vi "PSTR-Save Data.vi"(0 "Data in":T12, 1 "PSTR Params":T4={"Stimulus"={"Ear"=enum."Right", "BW (oct)"=0.25, "Seed"=37, "Ramp (ms)"=5.0, "On time (ms)"=300.0, "Off time (ms)"=300.0, "Delay (ms)"=10000.0}, "FreqSeq"={"Min (kHz)"=4.0, "Max (kHz)"=64.0, "Step (oct)"=0.5}, "LevelSeq"={"Min (dB)"=0.0, "Max (dB)"=80.0, "Step (dB)"=20.0}, "Seq"={"Order"=enum."Sequential", "Averages"=20}, "Response"={"Grass gain"=10000.0, "Window (ms)"=0.0}, "Hidden"={"Sample rate (Hz)"=200000.0, "Nfft"=0, "save raw"=FALSE, "sep"=0.0, "Window"=enum."NONE"}, "RejThr"=0.0}, 2 "Expt State":T1, 5 "path":path, 7 "CFTS-PSTR":T3, 11 "error in":errorcluster) -> (4 "Data out":T12, 8 "file path out":path, 15 "Error Out":errorcluster)   [LabVIEW 2020]
uses:
  Typedefs/PSTR-Data.ctl
  Typedefs/PSTR-Model Fit.ctl
  Typedefs/PSTR-Fit Parameters.ctl
  Typedefs/PSTR-Parameters.ctl
  Typedefs/PSTR-Stimulus Params.ctl
  Typedefs/PSTR-FreqSeq Params.ctl
  Typedefs/PSTR-LevelSeq Params.ctl
  Typedefs/PSTR-SeqParams.ctl
  Typedefs/PSTR-Response Params.ctl
  Typedefs/PSTR-Hidden Params.ctl
  Typedefs/PSTR-Window Shape.ctl
  Typedefs/PSTR-File Info.ctl
  CFTS VIs/CFTS-Experiment State.ctl
  CFTS VIs/CFTS-Globals.vi
panel:
  in  "Data":T2
  # "NF x NL x 2 x Npts"
  # "NF x NL x Npts"
  # "NF x NL"
  # "NF x NL x 2 x Npts"
  # "NF x NL x Npts"
  # "NF x NL"
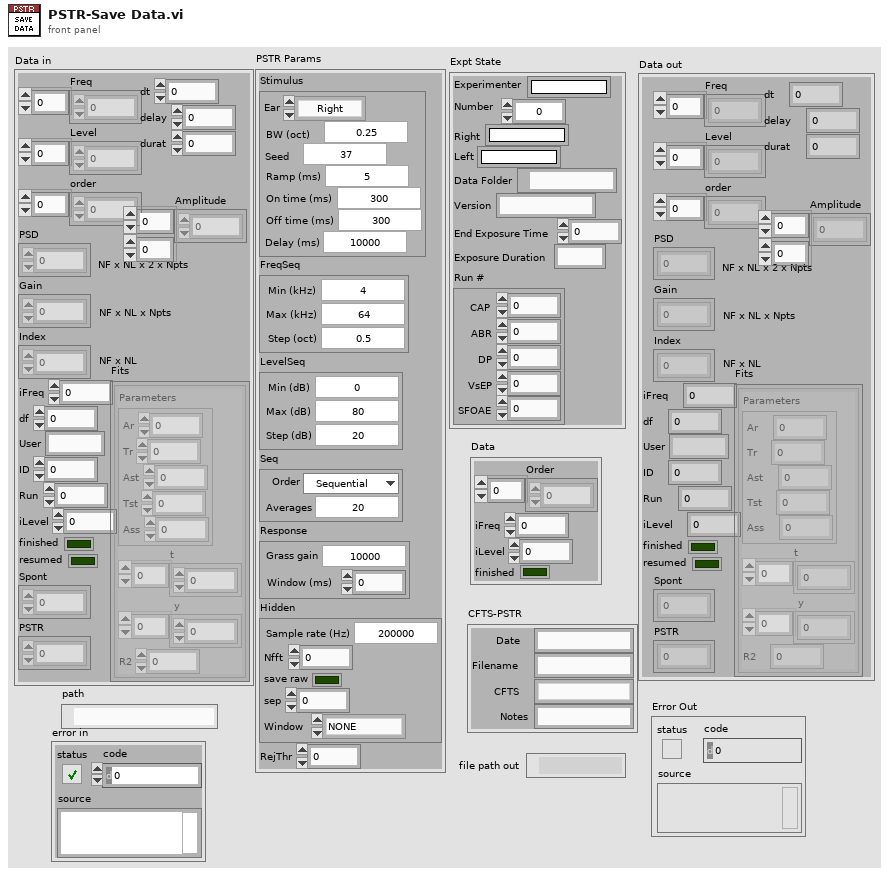
[diagram p1: front panel]
types:
  T1 = typedef "CFTS-Experiment State.ctl" = cluster{"Experimenter":string, "Number":u32, "Right":string, "Left":string, "Data Folder":path, "Version":string, "End Exposure Time":dbl, "Exposure Duration":string, "Run #":cluster{"CAP":i32, "ABR":i32, "DP":i32, "VsEP":i32, "SFOAE":i32}}
  T2 = cluster{"Order":i32[], "iFreq":i32, "iLevel":i32, "finished":bool}
  T3 = typedef "PSTR-File Info.ctl" = cluster{"Date":string, "Filename":string, "CFTS":string, "Notes":string}
  T4 = typedef "PSTR-Parameters.ctl" = cluster{"Stimulus":T5, "FreqSeq":T6, "LevelSeq":T7, "Seq":T8, "Response":T9, "Hidden":T10, "RejThr":dbl}
  T5 = typedef "PSTR-Stimulus Params.ctl" = cluster{"Ear":enum16{"Right", "Left"}, "BW (oct)":dbl, "Seed":i32, "Ramp (ms)":dbl, "On time (ms)":dbl, "Off time (ms)":dbl, "Delay (ms)":dbl}
  T6 = typedef "PSTR-FreqSeq Params.ctl" = cluster{"Min (kHz)":dbl, "Max (kHz)":dbl, "Step (oct)":dbl}
  T7 = typedef "PSTR-LevelSeq Params.ctl" = cluster{"Min (dB)":dbl, "Max (dB)":dbl, "Step (dB)":dbl}
  T8 = typedef "PSTR-SeqParams.ctl" = cluster{"Order":enum16{"Sequential", "Random"}, "Averages":i32}
  T9 = typedef "PSTR-Response Params.ctl" = cluster{"Grass gain":dbl, "Window (ms)":dbl}
  T10 = typedef "PSTR-Hidden Params.ctl" = cluster{"Sample rate (Hz)":dbl, "Nfft":i32, "save raw":bool, "sep":dbl, "Window":T11}
  T11 = typedef "PSTR-Window Shape.ctl" = enum16{"NONE", "Hamming"}
  T12 = typedef "PSTR-Data.ctl" = cluster{"Freq":dbl[], "Level":dbl[], "order":i32[], "PSD":dbl[][][][], "Gain":dbl[][][], "Index":dbl[][], "iFreq":i32, "df":dbl, "User":string, "ID":i32, "Run":i32, "iLevel":i32, "finished":bool, "resumed":bool, "Spont":dbl[][], "PSTR":dbl[][][], "dt":dbl, "delay":dbl, "durat":dbl, "Fits":T13[][], "Amplitude":dbl[][]}
  T13 = typedef "PSTR-Model Fit.ctl" = cluster{"Parameters":T14, "t":dbl[], "y":dbl[], "R2":dbl}
  T14 = typedef "PSTR-Fit Parameters.ctl" = cluster{"Ar":dbl, "Tr":dbl, "Ast":dbl, "Tst":dbl, "Ass":dbl}
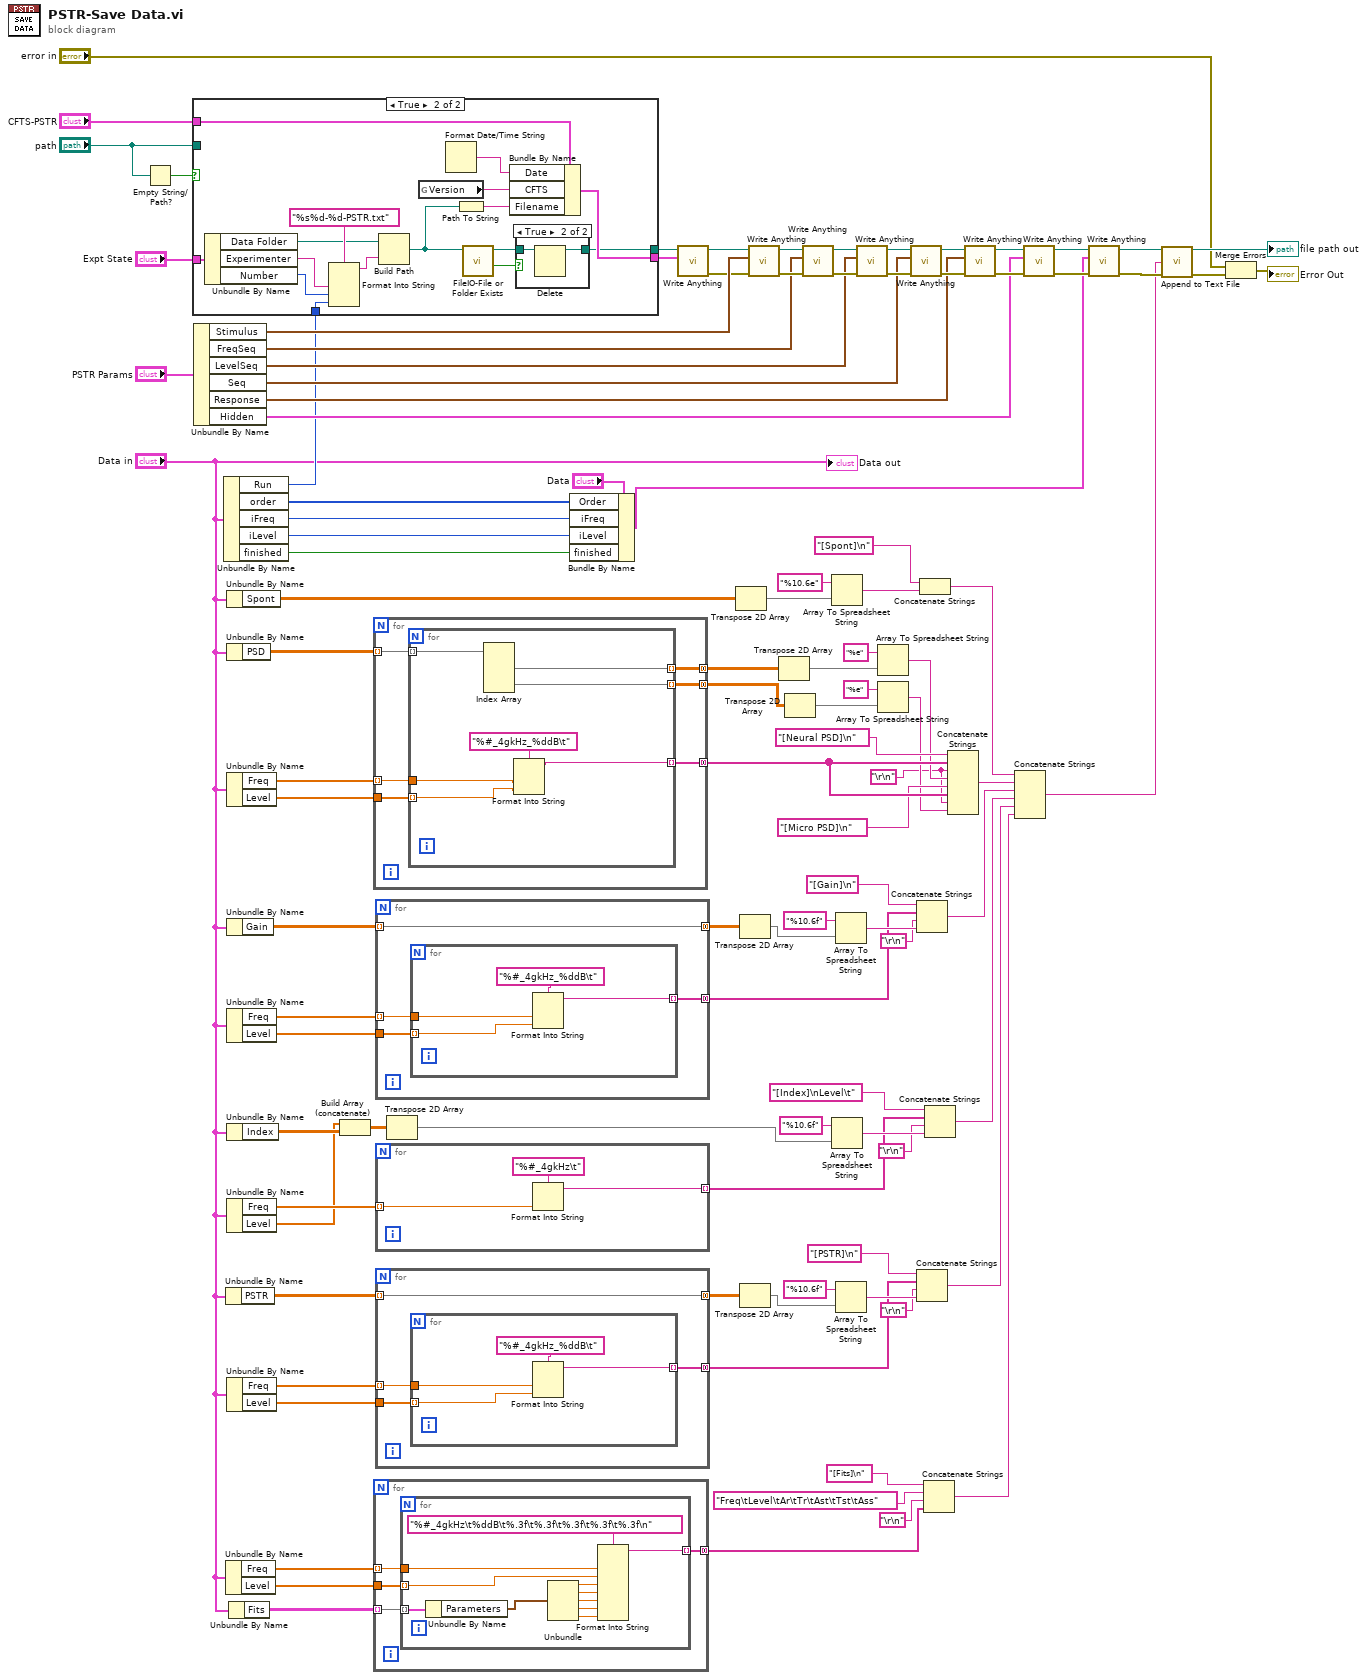
[diagram p0: block diagram]
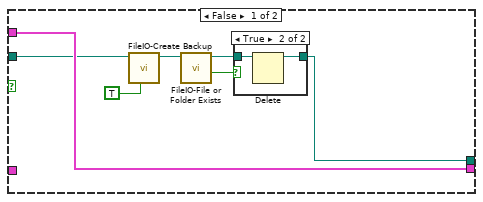
[diagram p2: hidden frame]
diagram:
  w34 = "\r\n"
  n1 = Empty String/Path?(string/path="path") -> (empty?=w5:bool)
  n2 = Unbundle By Name("PSTR Params") -> ("Stimulus"=w102:T5, "FreqSeq"=w92:T6, "LevelSeq"=w91:T7, "Seq"=w90:T8, "Response"=w89:T9, "Hidden"=w86:T10)
  n3 = Unbundle By Name("Data in") -> ("Run"=w35:i32, "order"=w63:i32[], "iFreq"=w37:i32, "iLevel"=w36:i32, "finished"=w33:bool)
  n4 = case shown="True" w5 {
    tunnel: "Expt State" -> [_ w131]
    tunnel: [w112 w123] -> w105
    tunnel: [w106 w119] -> w69
    tunnel: w35 -> [_ w118]
    tunnel: "path" -> [w111 _]
    tunnel: "CFTS-PSTR" -> [w112 w117]
    frame False {
      n5 = call "FileIO-Create Backup.vi"("Append date"=TRUE, "Path"=w111) -> ("Path (thru)"=w109:path)  [unwired: 6 in, 3 out]
      n6 = call "FileIO-File or Folder Exists.vi"("path"=w109) -> ("Exists?"=w107:bool, "dup path"=w108:path)  [unwired: 7 in, 2 out]
      n7 = case shown="True" w107 {
        tunnel: w108 -> [w113 w115]
        tunnel: [w113 w114] -> w106
        frame False {
        }
        frame True {
          n8 = Delete(path (use dialog)=w115) -> (deleted path=w114:path)  [unwired: 4 in, 2 out]
        }
      }
    }
    frame True {
      n9 = Unbundle By Name(w131) -> ("Data Folder"=w127:path, "Experimenter"=w130:string, "Number"=w129:u32)
      n10 = Format Into String(format string="%s%d-%d-PSTR.txt", w130, w129, w118) -> (resulting string=w126:string)  [unwired: 2 in, 1 out]
      n11 = Build Path(base path=w127, name or relative path=w126) -> (appended path=w122:path)
      n12 = global read "CFTS-Globals.vi" "Version"() -> (w116:string)
      n13 = Format Date/Time String() -> (date/time string=w124:string)  [unwired: 3 in]
      n14 = Path To String(path=w122) -> (string=w125:string)
      n15 = call "FileIO-File or Folder Exists.vi"("path"=w122) -> ("Exists?"=w121:bool, "dup path"=w120:path)  [unwired: 7 in, 2 out]
      n16 = Bundle By Name(cluster=w117, "Date"=w124, "CFTS"=w116, "Filename"=w125) -> (w123:T3)
      n17 = case shown="True" w121 {
        tunnel: w120 -> [w132 w134]
        tunnel: [w132 w133] -> w119
        frame False {
        }
        frame True {
          n18 = Delete(path (use dialog)=w134) -> (deleted path=w133:path)  [unwired: 4 in, 2 out]
        }
      }
    }
  }
  n19 = Unbundle By Name("Data in") -> ("PSTR"=w26:dbl[][][])
  n20 = Unbundle By Name("Data in") -> ("Freq"=w14:dbl[], "Level"=w13:dbl[])
  n21 = Unbundle By Name("Data in") -> ("Spont"=w28:dbl[][])
  n22 = Unbundle By Name("Data in") -> ("PSD"=w85:dbl[][][][])
  n23 = Unbundle By Name("Data in") -> ("Freq"=w84:dbl[], "Level"=w83:dbl[])
  n24 = Unbundle By Name("Data in") -> ("Gain"=w61:dbl[][][])
  n25 = Unbundle By Name("Data in") -> ("Freq"=w60:dbl[], "Level"=w59:dbl[])
  n26 = Unbundle By Name("Data in") -> ("Index"=w50:dbl[][])
  n27 = Unbundle By Name("Data in") -> ("Freq"=w49:dbl[], "Level"=w43:dbl[])
  n28 = Unbundle By Name("Data in") -> ("Freq"=w25:dbl[], "Level"=w24:dbl[])
  n29 = Unbundle By Name("Data in") -> ("Fits"=w15:T13[][])
  n30 = Build Array (concatenate)(w43, w50) -> (w42:dbl[][])
  n31 = for {
    tunnel: w85 -> [w140] mode=indexing
    tunnel: w84 -> [w139] mode=indexing
    tunnel: w83 -> [w138]
    tunnel: [w137] -> w80 mode=concatenating
    tunnel: [w136] -> w79 mode=concatenating
    tunnel: [w135] -> w74 mode=concatenating
    n32 = for {
      tunnel: w140 -> [w147] mode=indexing
      tunnel: w139 -> [w144]
      tunnel: w138 -> [w143] mode=indexing
      tunnel: [w142] -> w137 mode=indexing
      tunnel: [w146] -> w136 mode=indexing
      tunnel: [w145] -> w135 mode=indexing
      n33 = Index Array(array=w147) -> (element #1=w146:dbl[], element #2=w145:dbl[])  [unwired: 4 in]
      n34 = Format Into String(format string="%#_4gkHz_%ddB\t", w144, w143) -> (resulting string=w142:string)  [unwired: 2 in, 1 out]
    }
  }
  n35 = for {
    tunnel: w15 -> [w148] mode=indexing
    tunnel: w14 -> [w151] mode=indexing
    tunnel: w13 -> [w150]
    tunnel: [w149] -> w8 mode=concatenating
    n36 = for {
      tunnel: w151 -> [w162]
      tunnel: w150 -> [w160] mode=indexing
      tunnel: [w161] -> w149 mode=indexing
      tunnel: w148 -> [w159] mode=indexing
      n37 = Unbundle By Name(w159) -> ("Parameters"=w158:T14)
      n38 = Unbundle(w158) -> ("Ar"=w157:dbl, "Tr"=w156:dbl, "Ast"=w155:dbl, "Tst"=w154:dbl, "Ass"=w153:dbl)
      n39 = Format Into String(format string="%#_4gkHz\t%ddB\t%.3f\t%.3f\t%.3f\t%.3f\t%.3f\n", w162, w160, w157, w156, w155, w154, w153) -> (resulting string=w161:string)  [unwired: 2 in, 1 out]
    }
  }
  n40 = for {
    tunnel: w61 -> [w163] mode=indexing
    tunnel: w60 -> [w166] mode=indexing
    tunnel: w59 -> [w165]
    tunnel: [w164] -> w51 mode=concatenating
    tunnel: [w163] -> w58 mode=concatenating
    n41 = for {
      tunnel: w166 -> [w170]
      tunnel: w165 -> [w168] mode=indexing
      tunnel: [w169] -> w164 mode=indexing
      n42 = Format Into String(format string="%#_4gkHz_%ddB\t", w170, w168) -> (resulting string=w169:string)  [unwired: 2 in, 1 out]
    }
  }
  n43 = for {
    tunnel: w49 -> [w173] mode=indexing
    tunnel: [w171] -> w44 mode=indexing
    n44 = Format Into String(format string="%#_4gkHz\t", w173) -> (resulting string=w171:string)  [unwired: 2 in, 1 out]
  }
  n45 = for {
    tunnel: w26 -> [w174] mode=indexing
    tunnel: w25 -> [w177] mode=indexing
    tunnel: w24 -> [w176]
    tunnel: [w175] -> w18 mode=concatenating
    tunnel: [w174] -> w23 mode=concatenating
    n46 = for {
      tunnel: w177 -> [w181]
      tunnel: w176 -> [w179] mode=indexing
      tunnel: [w180] -> w175 mode=indexing
      n47 = Format Into String(format string="%#_4gkHz_%ddB\t", w181, w179) -> (resulting string=w180:string)  [unwired: 2 in, 1 out]
    }
  }
  n48 = Transpose 2D Array(2D array=w42) -> (transposed array=w41:dbl[][])
  n49 = Bundle By Name(cluster="Data", "Order"=w63, "iFreq"=w37, "iLevel"=w36, "finished"=w33) -> (w62:T2)
  n50 = call "Write Anything.vi"("Anything"=w105, "Path (dialog)"=w69) -> ("Error Out"=w101:errorcluster, "Path out"=w104:path)  [unwired: 8 in]
  n51 = Transpose 2D Array(2D array=w28) -> (transposed array=w31:dbl[][])
  n52 = Transpose 2D Array(2D array=w58) -> (transposed array=w56:dbl[][])
  n53 = Transpose 2D Array(2D array=w23) -> (transposed array=w21:dbl[][])
  n54 = call "Write Anything.vi"("Error In"=w101, "Anything"=w102, "Path (dialog)"=w104) -> ("Error Out"=w96:errorcluster, "Path out"=w100:path)  [unwired: 7 in]
  n55 = Transpose 2D Array(2D array=w79) -> (transposed array=w71:dbl[][])
  n56 = Transpose 2D Array(2D array=w74) -> (transposed array=w70:dbl[][])
  n57 = call "Write Anything.vi"("Error In"=w96, "Anything"=w92, "Path (dialog)"=w100) -> ("Error Out"=w95:errorcluster, "Path out"=w99:path)  [unwired: 7 in]
  n58 = Array To Spreadsheet String(array=w31, 3:"%10.6e" ("format string")) -> (spreadsheet string=w30:string)  [unwired: 1 in]
  n59 = Array To Spreadsheet String(array=w41, 3:"%10.6f" ("format string")) -> (spreadsheet string=w47:string)  [unwired: 1 in]
  n60 = Array To Spreadsheet String(array=w56, 3:"%10.6f" ("format string")) -> (spreadsheet string=w54:string)  [unwired: 1 in]
  n61 = Array To Spreadsheet String(array=w21, 3:"%10.6f" ("format string")) -> (spreadsheet string=w20:string)  [unwired: 1 in]
  n62 = call "Write Anything.vi"("Error In"=w95, "Anything"=w91, "Path (dialog)"=w99) -> ("Error Out"=w94:errorcluster, "Path out"=w98:path)  [unwired: 7 in]
  n63 = Array To Spreadsheet String(array=w71, 3:"%e" ("format string")) -> (spreadsheet string=w76:string)  [unwired: 1 in]
  n64 = Array To Spreadsheet String(array=w70, 3:"%e" ("format string")) -> (spreadsheet string=w73:string)  [unwired: 1 in]
  n65 = call "Write Anything.vi"("Error In"=w94, "Anything"=w90, "Path (dialog)"=w98) -> ("Error Out"=w93:errorcluster, "Path out"=w97:path)  [unwired: 7 in]
  n66 = Concatenate Strings("[Gain]\n", w51, "\r\n", w54) -> (w52:string)
  n67 = Concatenate Strings("[PSTR]\n", w18, "\r\n", w20) -> (w16:string)
  n68 = Concatenate Strings("[Spont]\n", w30) -> (w29:string)
  n69 = Concatenate Strings("[Fits]\n", "Freq\tLevel\tAr\tTr\tAst\tTst\tAss" ("format string"), "\r\n", w8) -> (w9:string)
  n70 = Concatenate Strings("[Index]\nLevel\t", w44, "\r\n", w47) -> (w45:string)
  n71 = Concatenate Strings("[Neural PSD]\n", w80, w34, w76, "[Micro PSD]\n", w80, w34, w73) -> (w72:string)
  n72 = call "Write Anything.vi"("Error In"=w93, "Anything"=w89, "Path (dialog)"=w97) -> ("Error Out"=w87:errorcluster, "Path out"=w88:path)  [unwired: 7 in]
  n73 = Concatenate Strings(w29, w72, w52, w45, w16, w9) -> (w55:string)
  n74 = call "Write Anything.vi"("Error In"=w87, "Anything"=w86, "Path (dialog)"=w88) -> ("Error Out"=w68:errorcluster, "Path out"=w67:path)  [unwired: 7 in]
  n75 = call "Write Anything.vi"("Error In"=w68, "Anything"=w62, "Path (dialog)"=w67) -> ("Error Out"=w65:errorcluster, "Path out"=w66:path)  [unwired: 7 in]
  n76 = call "Append to Text File.vi"("file path"=w66, "text"=w55, "error in (no error)"=w65) -> ("file path out"=→"file path out":path, "error out"=w81:errorcluster)  [unwired: 11 in]
  n77 = Merge Errors("error in", w81) -> (→"Error Out":errorcluster)
  "Data out" <- "Data in"
